vi "close.vi"(8 "error in":errorcluster, 11 "testmod runtime in":refnum<class "testmod runtime.lvclass">) -> (0 "error out":errorcluster)   [LabVIEW 2013, in "testmod runtime.lvclass"]
doc: "Provides an interface for terminating a module instance. While this interface performs no operations, a child should close and deallocate any open references or memory."
uses:
  testmod runtime.lvclass
  testmod runtime.lvclass/testmod runtime.ctl
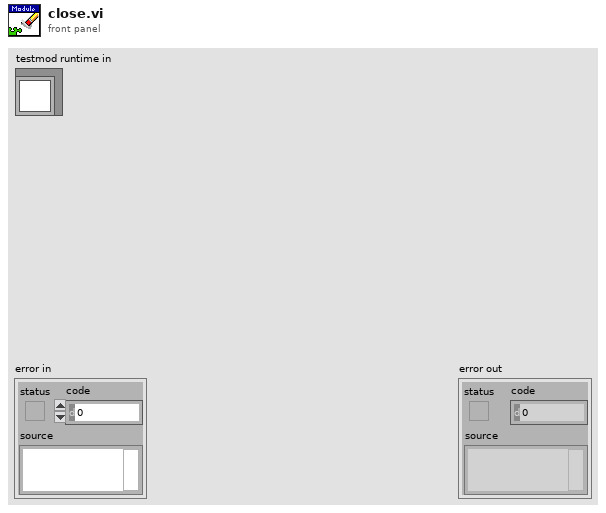
[diagram p1: front panel]
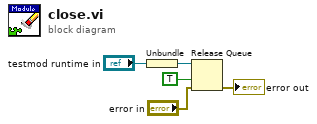
[diagram p0: block diagram]
diagram:
  n1 = Unbundle("testmod runtime in") -> (w4:refnum<queue>)
  n2 = Release Queue(queue=w4, force destroy? (F)=TRUE, error in (no error)="error in") -> (error out=→"error out":errorcluster)  [unwired: 2 out]
